vi "Close DSF Configuration Data.vi"(6 "version (no change)":T1, 8 "error in (no error)":errorcluster, 10 "write file if changed (T)":bool=TRUE, 11 "Configuration Session":refnum<class "Configuration.lvclass">) -> (0 "error out":errorcluster, 3 "file path":path)   [LabVIEW 2017, in "DSF Core.lvlib" / "Configuration.lvclass"]
doc: "Writes data to the platform-independent configuration file identified by <B>dsf refnum</B> and then closes the reference to that file."
uses:
  Configuration.lvclass
  Typedefs/DSF Version Info.ctl
  Configuration.lvclass/Configuration.ctl
  DSF Core.lvlib
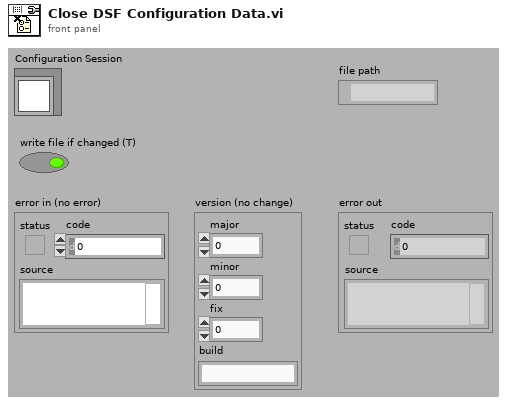
[diagram p1: front panel]
types:
  T1 = typedef "DSF Core.lvlib/DSF Version Info.ctl" = cluster{"major":u32, "minor":u32, "fix":u32, "build":string}
  T2 = typedef "DSF Core.lvlib/Configuration.lvclass/DSF Config Data Ref.ctl" = refnum<data-value>
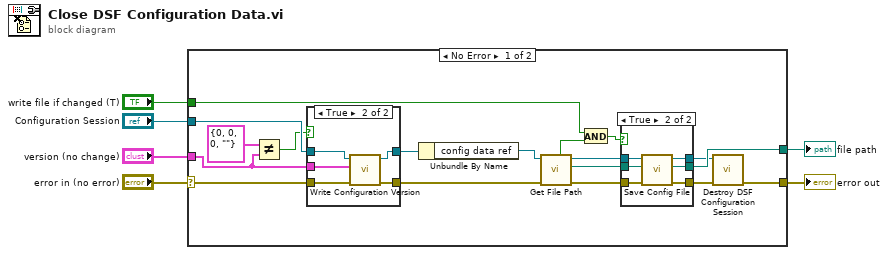
[diagram p0: block diagram]
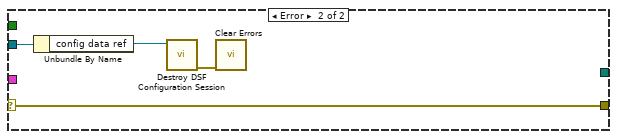
[diagram p4: hidden frame]
diagram:
  n1 = case shown="No Error" "error in (no error)" {
    selector: "error in (no error)" -> [w23 w44]
    tunnel: "Configuration Session" -> [w19 w42]
    tunnel: "write file if changed (T)" -> [w24 _]
    tunnel: [w22 w44] -> w4
    tunnel: [w21 _] -> w3
    tunnel: "version (no change)" -> [w16 _]
    frame No Error {
      n2 = Not Equal?(x=T1 {"major"=0, "minor"=0, "fix"=0, "build"=""} ("version"), y=w16) -> (x != y?=w17:bool)
      n3 = case shown="True" w17 {
        tunnel: w23 -> [w25 w31]
        tunnel: [w25 w30] -> w20
        tunnel: w19 -> [w26 w29]
        tunnel: [w26 w28] -> w15
        tunnel: w16 -> [_ w27]
        frame False {
        }
        frame True {
          n4 = call "Write Configuration Version.vi"("error in (no error)"=w31, "Configuration Version"=w27, "Configuration Session in"=w29) -> ("error out"=w30:errorcluster, "Configuration Session out"=w28:refnum<class "Configuration.lvclass">)  [unwired: 7 in]
        }
      }
      n5 = Unbundle By Name(w15) -> ("config data ref"=w7:T2)
      n6 = call "Get File Path.vi"("error in (no error)"=w20, "DSF Configuration Reference in"=w7) -> ("error out"=w9:errorcluster, "file path"=w8:path, "DSF Configuration Reference out"=w13:T2, "need update"=w10:bool)  [unwired: 1 in, 5 out]
      n7 = And(x=w24, y=w10) -> (x .and. y?=w14:bool)
      n8 = case shown="True" w14 {
        tunnel: w9 -> [w34 w40]
        tunnel: w13 -> [w33 w35]
        tunnel: [w34 w39] -> w11
        tunnel: [w33 w38] -> w12
        tunnel: w8 -> [w32 w37]
        tunnel: [w32 w36] -> w21
        frame False {
        }
        frame True {
          n9 = call "Save Config File.vi"("error in (no error)"=w40, "file path"=w37, "DSF Configuration Reference in"=w35) -> ("error out"=w39:errorcluster, "file path out"=w36:path, "DSF Configuration Reference out"=w38:T2)  [unwired: 6 out]
        }
      }
      n10 = call "Destroy DSF Configuration Session.vi"("error in (no error)"=w11, "config data ref"=w12) -> ("error out"=w22:errorcluster)  [unwired: 9 in]
    }
    frame Error {
      n11 = Unbundle By Name(w42) -> ("config data ref"=w41:T2)
      n12 = call "Destroy DSF Configuration Session.vi"("config data ref"=w41) -> ("error out"=w43:errorcluster)  [unwired: 10 in]
      n13 = call <vilib>:"Clear Errors.vi"("error in (no error)"=w43) -> ()  [unwired: 5 in, 2 out]
    }
  }
  "error out" <- w4
  "file path" <- w3
